vi "Check Stop Message.vi"(8 "error in (no error)":errorcluster, 11 "rfsa queue":refnum<queue>) -> (0 "error out":errorcluster, 3 "stop?":bool)   [LabVIEW 2021]
uses:
  Messaging/RFSA Message.ctl
  RFSA Configuration.ctl
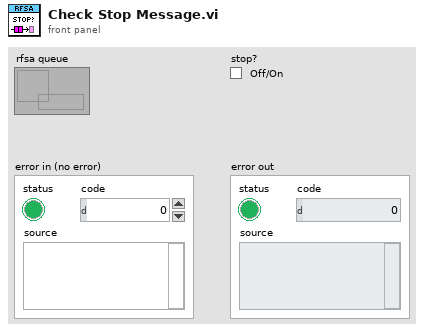
[diagram p1: front panel]
types:
  T1 = typedef "RFSA Message.ctl" = enum16{"Initialize RF", "Run RF", "Stop RF", "Exit"}
  T2 = typedef "RFSA Configuration.ctl" = cluster{"rfsa ref":refnum<k15>, "cent freq":dbl, "iq rate":dbl, "power":dbl, "N/block":i64, "msg":T1}
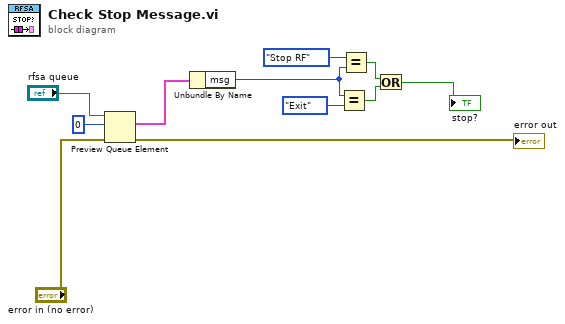
[diagram p0: block diagram]
diagram:
  n1 = Preview Queue Element(queue="rfsa queue", timeout in ms (-1)=0, error in (no error)="error in (no error)") -> (element=w6:T2, error out=→"error out":errorcluster)  [unwired: 2 out]
  n2 = Unbundle By Name(w6) -> ("msg"=w5:T1)
  n3 = Equal?(x=w5, y=RFSA_Message."Exit") -> (x = y?=w4:bool)
  n4 = Equal?(x=RFSA_Message."Stop RF", y=w5) -> (x = y?=w3:bool)
  n5 = Or(x=w3, y=w4) -> (x .or. y?=→"stop?":bool)
